vi "test_33600A.vi"() -> ()   [LabVIEW 2020]
uses:
  General AC source/Type definitions/AC Source type.ctl
  General AC source/Type definitions/AC Source.ctl
  external libraries/AWG/Agilent 3352X Series/Agilent 3352X Series.lvlib
  external libraries/AWG/Agilent 33XXX Series/Agilent 33XXX Series.lvlib
panel:
  out "Interface Information:Interface Type":u16(ring)=1 items=["GPIB"=1, "VXI"=2, "GPIB-VXI"=3, "Serial"=4, "PXI"=5, "TCPIP"=6, "USB"=7, "FireWire"=9]
  out "read buffer system error":string
  out "read buffer":string
  out "idn string":string
  out "error out":errorcluster
  out "Init status":string
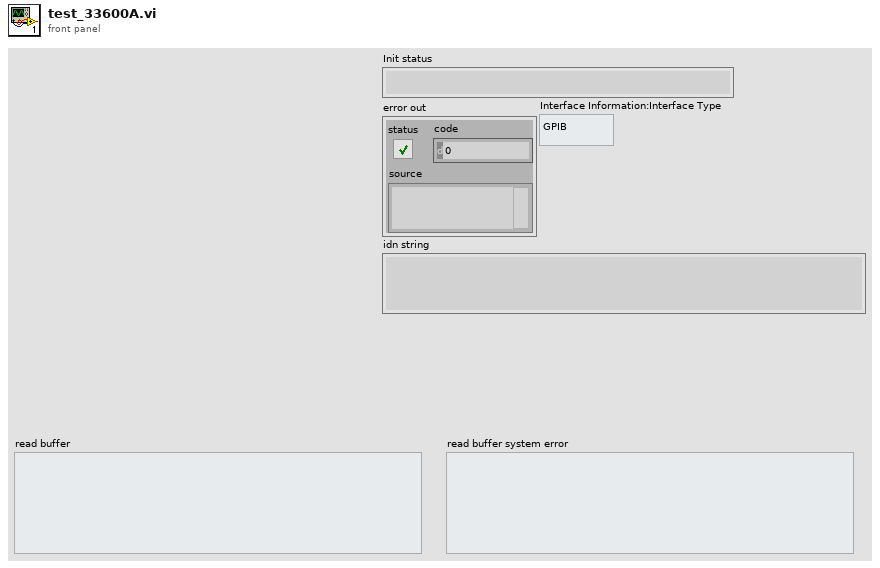
[diagram p1: front panel]
types:
  T1 = typedef "AC Source.ctl" = cluster{"AC Source type":T2, "VISA":refnum<visa-resource-name>, "Ref. clock (Hz)":dbl, "status ref":refnum<vi>, "Fluke 57XX wideband output":bool, "Fluke 57XX ignore errors":bool, "Synchronization by AC signal":bool}
  T2 = typedef "AC Source type.ctl" = enum16{"Fluke 5XXX calibrator", "Tektronix AFG3000 series", "dummy", "Agilent 331xxA to 332xxA", "Agilent 335xxA to 336xxA"}
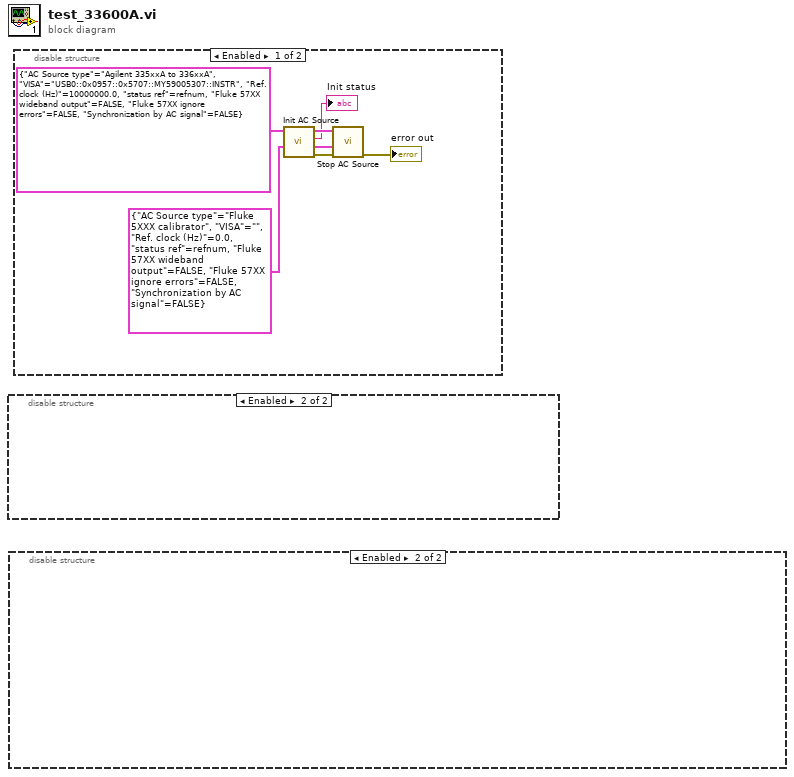
[diagram p0: block diagram]
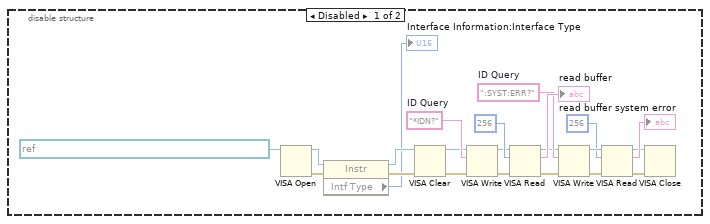
[diagram p2: hidden frame]
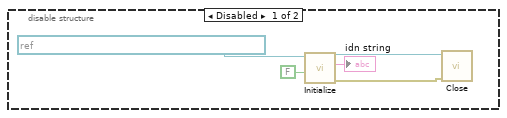
[diagram p3: hidden frame]
diagram:
  n1 = disable-structure shown="Enabled" {
    frame Disabled {
      n2 = call "Initialize.vi"("Reset (Enable)"=FALSE, "VISA resource name"=refnum<visa-resource-name> "USB0::0x0957::0x5707::MY59005307::INSTR") -> ("error out"=w4:errorcluster, "idn string"=→"idn string":string, "VISA resource name out"=w3:refnum<visa-resource-name>)  [unwired: 7 in]
      n3 = call "Close.vi"("error in (no error)"=w4, "VISA resource name"=w3) -> ()  [unwired: 9 in, 1 out]
    }
    frame Enabled {
    }
  }
  n4 = disable-structure shown="Enabled" {
    frame Disabled {
      w15 = ":SYST:ERR?"  # ID Query
      w26 = "*IDN?"  # ID Query
      n5 = VISA Open(VISA resource name=refnum<visa-resource-name> "USB0::0x0957::0x5707::MY59005307::INSTR") -> (VISA resource name=w10:refnum<visa-resource-name>, error out=w9:errorcluster)  [unwired: 2 in, 2 out]
      n6 = property class="Instr"(reference=w10, error in=w9) -> (reference out=w7:refnum<visa-resource-name>, error out=w8:errorcluster, "Intf Type"=→"Interface Information:Interface Type":u16)
      n7 = VISA Clear(VISA resource name=w7, error in (no error)=w8) -> (VISA resource name out=w22:refnum<visa-resource-name>, error out=w21:errorcluster)
      n8 = VISA Write(VISA resource name=w22, write buffer=w26, error in (no error)=w21) -> (VISA resource name out=w23:refnum<visa-resource-name>, error out=w24:errorcluster)  [unwired: 1 out]
      n9 = VISA Read(VISA resource name=w23, byte count=u32 256, error in (no error)=w24) -> (VISA resource name out=w13:refnum<visa-resource-name>, read buffer=→"read buffer":string, error out=w14:errorcluster)  [unwired: 1 out]
      n10 = VISA Write(VISA resource name=w13, write buffer=w15, error in (no error)=w14) -> (VISA resource name out=w18:refnum<visa-resource-name>, error out=w17:errorcluster)  [unwired: 1 out]
      n11 = VISA Read(VISA resource name=w18, byte count=u32 256, error in (no error)=w17) -> (VISA resource name out=w11:refnum<visa-resource-name>, read buffer=→"read buffer system error":string, error out=w12:errorcluster)  [unwired: 1 out]
      n12 = VISA Close(VISA resource name=w11, error in (no error)=w12) -> ()  [unwired: 1 out]
    }
    frame Enabled {
    }
  }
  n13 = disable-structure shown="Enabled" {
    frame Enabled {
      n14 = call "Init AC Source.vi"("AC sync source"=T1 {"AC Source type"=enum."Fluke 5XXX calibrator", "VISA"="", "Ref. clock (Hz)"=0.0, "status ref"=refnum, "Fluke 57XX wideband output"=FALSE, "Fluke 57XX ignore errors"=FALSE, "Synchronization by AC signal"=FALSE}, "AC source"=T1 {"AC Source type"=enum."Agilent 335xxA to 336xxA", "VISA"="USB0::0x0957::0x5707::MY59005307::INSTR", "Ref. clock (Hz)"=10000000.0, "status ref"=refnum, "Fluke 57XX wideband output"=FALSE, "Fluke 57XX ignore errors"=FALSE, "Synchronization by AC signal"=FALSE}) -> ("error out"=w34:errorcluster, "AC sync source out"=w28:T1, "Init status"=→"Init status":string, "AC source out"=w33:T1)  [unwired: 6 in]
      n15 = call "Stop AC Source.vi"("error in (no error)"=w34, "AC sync source"=w28, "AC source"=w33) -> ("error out"=→"error out":errorcluster)  [unwired: 6 in, 2 out]
    }
    frame Disabled {
    }
  }
